vi "Warn Deprecated.vi"(8 "error in (no error)":errorcluster, 9 "replacement":string, 10 "deprecated version":string, 11 "name":string) -> (0 "error out":errorcluster)   [LabVIEW 2013, in "libssh2.lvlib"]
uses:
  libssh2.lvlib
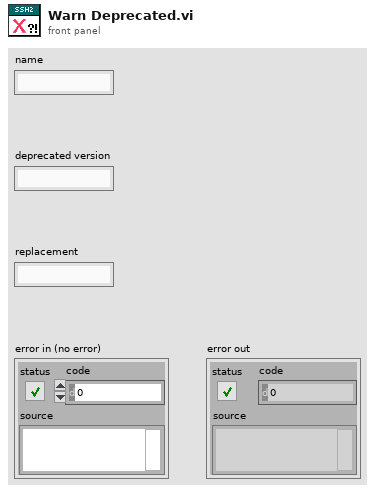
[diagram p1: front panel]
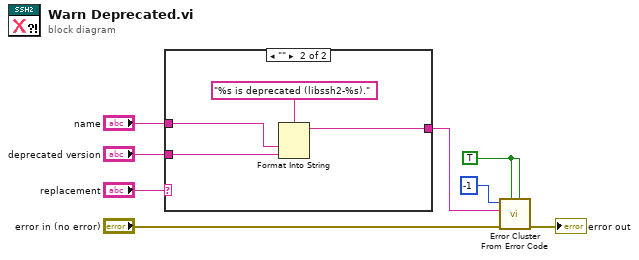
[diagram p0: block diagram]
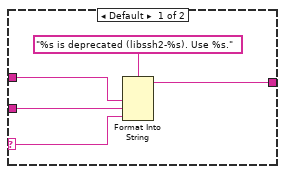
[diagram p2: hidden frame]
diagram:
  w6 = TRUE ("show call chain? (False)")
  n1 = case shown="\"\"" "replacement" {
    selector: "replacement" -> [w9 _]
    tunnel: "deprecated version" -> [w12 w16]
    tunnel: [w11 w15] -> w3
    tunnel: "name" -> [w10 w14]
    frame Default {
      n2 = Format Into String(format string="%s is deprecated (libssh2-%s). Use %s." ("error message (\"\")"), w10, w12, w9) -> (resulting string=w11:string)  [unwired: 2 in, 1 out]
    }
    frame "" {
      n3 = Format Into String(format string="%s is deprecated (libssh2-%s)." ("error message (\"\")"), w14, w16) -> (resulting string=w15:string)  [unwired: 2 in, 1 out]
    }
  }
  n4 = call <vilib>:"Error Cluster From Error Code.vi"("is warning? (False)"=w6, "show call chain? (False)"=w6, "error in (no error)"="error in (no error)", "error message (\"\")"=w3, "error code (0)"=-1) -> ("error out"=→"error out":errorcluster)  [unwired: 4 in]
